vi "DN4_2Darray1DWfm.vi"(3 "rate":dbl, 4 "StartTime":timestamp, 5 "2D Array":dbl[][](array[numeric])) -> (0 "EndTime":timestamp, 1 "1D Wfm":waveform(dbl)[](array[waveform]))   [LabVIEW 2020]
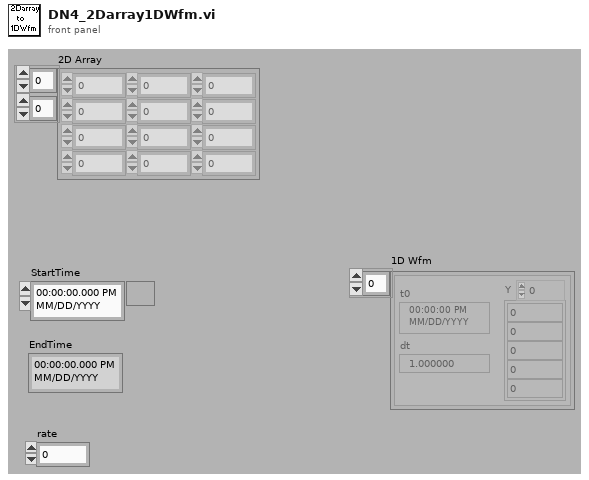
[diagram p1: front panel]
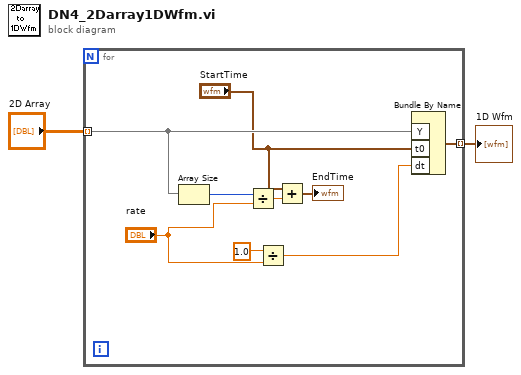
[diagram p0: block diagram]
diagram:
  n1 = for {
    tunnel: "2D Array" -> [w9] mode=indexing
    tunnel: [w11] -> w1 mode=indexing
    n2 = Array Size(array=w9) -> (size(s)=w8:i32)
    n3 = Divide(x=w8, y="rate") -> (x/y=w5:dbl)
    n4 = Divide(x=1.0, y="rate") -> (x/y=w7:dbl)
    n5 = Add(x="StartTime", y=w5) -> (x+y=→"EndTime":timestamp)
    n6 = Bundle By Name("Y"=w9, "t0"="StartTime", "dt"=w7) -> (w11:waveform(dbl))  [unwired: 1 out]
  }
  "1D Wfm" <- w1
